vi "display.vi"() -> ()   [LabVIEW 2018]
panel:
  out "element":string
  out "Display":string[][](table)
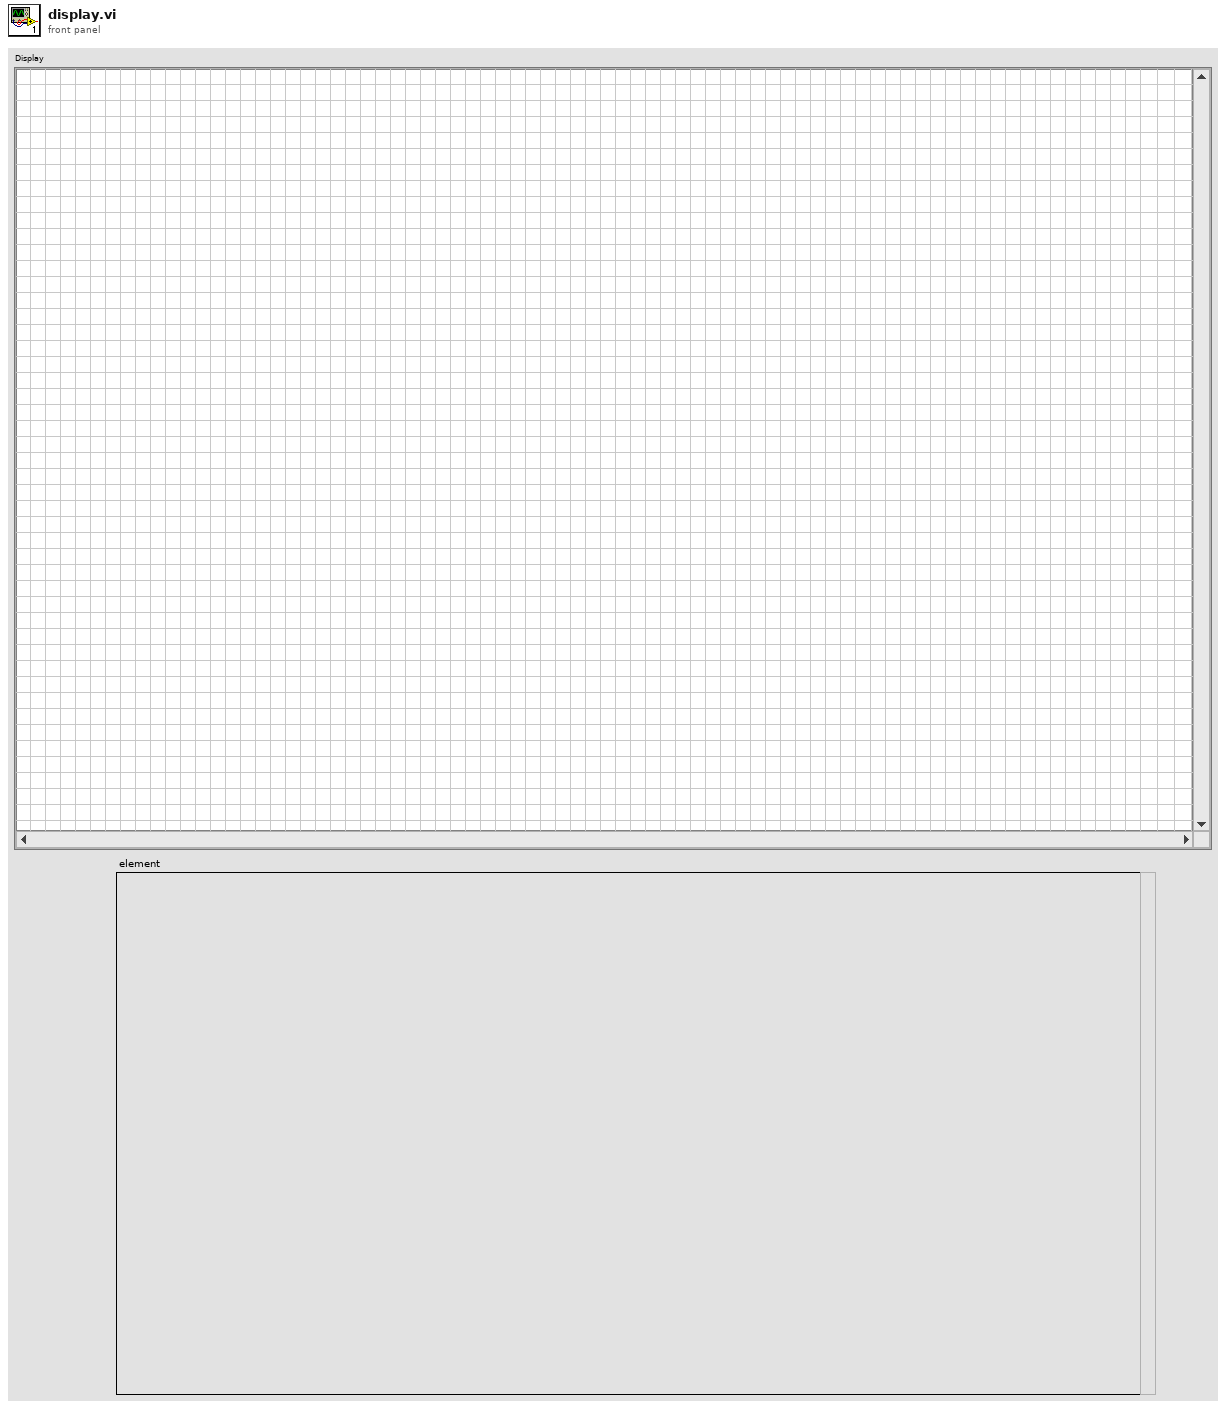
[diagram p1: front panel]
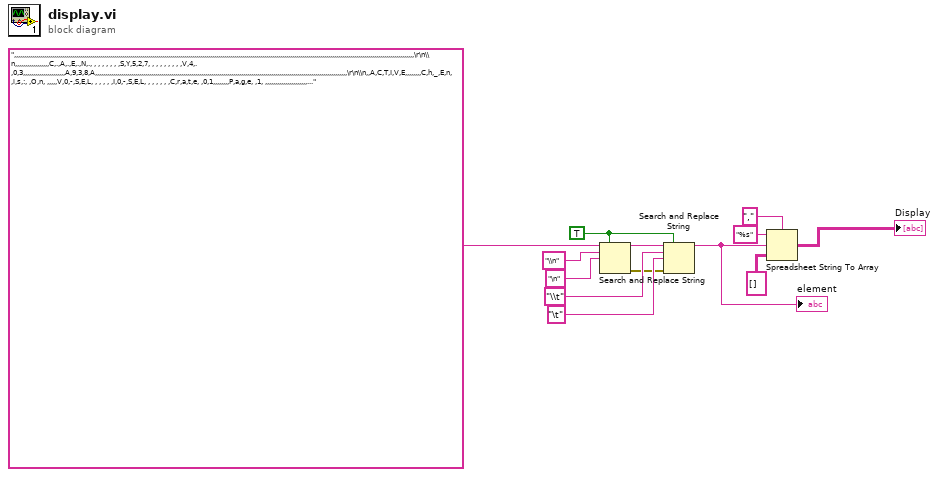
[diagram p0: block diagram]
diagram:
  w2 = TRUE ("replace all? (F)")
  n1 = Search and Replace String(replace all?=w2, input string=",,,,,,,,,,,,,,,,,,,,,,,,,,,,,,,,,,,,,,,,,,,,,,,,,,,,,,,,,,,,,,,,,,,,,,,,,,,,,,,,,,,,,,,,,,,,,,,,,,,,,,,,,,,,,,,,,,,,,,,,,,,,,,,,,,,,,,,,,,,,,,,,,,,,,,,,,,,,,,,,,,,,,,,,,,,,,,,,,,,,,,,,,,,,,,,,,,,,,,,,\r\n\\n,,,,,,,,,,,,,,,,,C,.,A,.,E,.,N,., , , , , , , ,S,Y,5,2,7, , , , , , , , ,V,4,.,0,3,,,,,,,,,,,,,,,,,,,,,A,9,3,8,A,,,,,,,,,,,,,,,,,,,,,,,,,,,,,,,,,,,,,,,,,,,,,,,,,,,,,,,,,,,,,,,,,,,,,,,,,,,,,,,,,,,,,,,,,,,,,,,,,,,,,,,,,,,,,,,,,,,,,,,,,,,,,,\r\n\\n,,A,C,T,I,V,E,,,,,,,,C,h,_,E,n, ,i,s,:, ,O,n, ,,,,,V,0,-,S,E,L, , , , , ,I,0,-,S,E,L, , , , , , ,C,r,a,t,e, ,0,1,,,,,,,,P,a,g,e, ,1, ,,,,,,,,,,,,,,,,,,,,,,,,,,,,,,,,,,,,,,,,,,,,,,,,,,,,,,,,,,,,,,,,,,,,,,,,,,,,,,,,,,,,,,,,,,,,,,,,,,,,,,,,,,,,,,,,,,,,,,,,,,,,\r\n\\n,,,,,,,,,,,,,,,,,,,,,,,,,,,,,,,,,,,,,,,,,,,,,,,,,,,,,,,,,,,,,,,,,,,,,,,,,,,,,,,,,,,,,,,,,,,,,,,,,,,,,,,,,,,,,,,,,,,,,,,,,,,,,,,,,,,,,,,,,,,,,,,,,,,,,,,,,,,,,,,,,,,,,,,,,,,,,,,,,,,,,,,,,,,,,,,,,,,,,,,,\r\n\\n, ,C,h,a,n,n,e,l, , , , , ,S,V,m,a,x, , ,R,u,p, , ,R,d,w,n, , ,T,r,i,p, ,T,r,i,p,E,x, ,P,r,O,n, ,P,r,O,f,f, ,P,o,n, , ,P,d,w,n, ,P,s,w,d, ,O,n,/,O,f,f, , ,C,h,#,,,,,,,,,,,,,,,,,,,,,,,,,,,,,,,,,,,,,,,,,,,,,,,,,,,,,,,,,,,,,,,,,,,,,,,,,,,,,,,,,,,,,,,,,,,,,,,,,,,,,,,,,,,,,,,,,,,,,,,,\r\n\\n, ,C,H,A,N,N,E,L,1,6, , , , ,2,0,0,0, , ,1,0,0, , ,1,0,0, , ,0,1,0,.,0, , , ,-,-, , , , ,0,1, , , ,0,1, , , ,O,f,f, , ,R,d,w,n, , , , , , , , , , , , , ,1,.,1,6,,,,,,,,,,,,,,,,,,,,,,,,,,,,,,,,,,,,,,,,,,,,,,,,,,,,,,,,,,,,,,,,,,,,,,,,,,,,,,,,,,,,,,,,,,,,,,,,,,,,,,,,,,,,,,,,,,,,,,,,\r\n\\n, ,C,H,A,N,N,E,L,1,7, , , , ,2,0,0,0, , ,1,0,0, , ,1,0,0, , ,0,1,0,.,0, , , ,-,-, , , , ,0,1, , , ,0,1, , , ,O,f,f, , ,R,d,w,n, , , , , , , , , , , , , ,1,.,1,7,,,,,,,,,,,,,,,,,,,,,,,,,,,,,,,,,,,,,,,,,,,,,,,,,,,,,,,,,,,,,,,,,,,,,,,,,,,,,,,,,,,,,,,,,,,,,,,,,,,,,,,,,,,,,,,,,,,,,,,,\r\n\\n, ,C,H,A,N,N,E,L,1,8, , , , ,2,0,0,0, , ,1,0,0, , ,1,0,0, , ,0,1,0,.,0, , , ,-,-, , , , ,0,1, , , ,0,1, , , ,O,f,f, , ,R,d,w,n, , , , , , , , , , , , , ,1,.,1,8,,,,,,,,,,,,,,,,,,,,,,,,,,,,,,,,,,,,,,,,,,,,,,,,,,,,,,,,,,,,,,,,,,,,,,,,,,,,,,,,,,,,,,,,,,,,,,,,,,,,,,,,,,,,,,,,,,,,,,,,\r\n\\n, ,C,H,A,N,N,E,L,1,9, , , , ,2,0,0,0, , ,1,0,0, , ,1,0,0, , ,0,1,0,.,0, , , ,-,-, , , , ,0,1, , , ,0,1, , , ,O,f,f, , ,R,d,w,n, , , , , , , , , , , , , ,1,.,1,9,,,,,,,,,,,,,,,,,,,,,,,,,,,,,,,,,,,,,,,,,,,,,,,,,,,,,,,,,,,,,,,,,,,,,,,,,,,,,,,,,,,,,,,,,,,,,,,,,,,,,,,,,,,,,,,,,,,,,,,,\r\n\\n, ,C,H,A,N,N,E,L,2,0, , , , ,2,0,0,0, , ,1,0,0, , ,1,0,0, , ,0,1,0,.,0, , , ,-,-, , , , ,0,1, , , ,0,1, , , ,O,f,f, , ,R,d,w,n, , , , , , , , , , , , , ,1,.,2,0,,,,,,,,,,,,,,,,,,,,,,,,,,,,,,,,,,,,,,,,,,,,,,,,,,,,,,,,,,,,,,,,,,,,,,,,,,,,,,,,,,,,,,,,,,,,,,,,,,,,,,,,,,,,,,,,,,,,,,,,\r\n\\n, ,C,H,A,N,N,E,L,2,1, , , , ,2,0,0,0, , ,1,0,0, , ,1,0,0, , ,0,1,0,.,0, , , ,-,-, , , , ,0,1, , , ,0,1, , , ,O,f,f, , ,R,d,w,n, , , , , , , , , , , , , ,1,.,2,1,,,,,,,,,,,,,,,,,,,,,,,,,,,,,,,,,,,,,,,,,,,,,,,,,,,,,,,,,,,,,,,,,,,,,,,,,,,,,,,,,,,,,,,,,,,,,,,,,,,,,,,,,,,,,,,,,,,,,,,,\r\n\\n, ,C,H,A,N,N,E,L,2,2, , , , ,2,0,0,0, , ,1,0,0, , ,1,0,0, , ,0,1,0,.,0, , , ,-,-, , , , ,0,1, , , ,0,1, , , ,O,f,f, , ,R,d,w,n, , , , , , , , , , , , , ,1,.,2,2,,,,,,,,,,,,,,,,,,,,,,,,,,,,,,,,,,,,,,,,,,,,,,,,,,,,,,,,,,,,,,,,,,,,,,,,,,,,,,,,,,,,,,,,,,,,,,,,,,,,,,,,,,,,,,,,,,,,,,,,\r\n\\n, ,C,H,A,N,N,E,L,2,3, , , , ,2,0,0,0, , ,1,0,0, , ,1,0,0, , ,0,1,0,.,0, , , ,-,-, , , , ,0,1, , , ,0,1, , , ,O,f,f, , ,R,d,w,n, , , , , , , , , , , , , ,1,.,2,3,,,,,,,,,,,,,,,,,,,,,,,,,,,,,,,,,,,,,,,,,,,,,,,,,,,,,,,,,,,,,,,,,,,,,,,,,,,,,,,,,,,,,,,,,,,,,,,,,,,,,,,,,,,,,,,,,,,,,,,,\r\n\\n, ,C,H,A,N,N,E,L,2,4, , , , ,2,0,0,0, , ,1,0,0, , ,1,0,0, , ,0,1,0,.,0, , , ,-,-, , , , ,0,1, , , ,0,1, , , ,O,f,f, , ,R,d,w,n, , , , , , , , , , , , , ,1,.,2,4,,,,,,,,,,,,,,,,,,,,,,,,,,,,,,,,,,,,,,,,,,,,,,,,,,,,,,,,,,,,,,,,,,,,,,,,,,,,,,,,,,,,,,,,,,,,,,,,,,,,,,,,,,,,,,,,,,,,,,,,\r\n\\n, ,C,H,A,N,N,E,L,0,0, , , , ,2,0,0,0, , ,1,0,0, , ,1,0,0, , ,0,1,0,.,0, , , ,-,-, , , , ,0,1, , , ,0,1, , , ,O,f,f, , ,R,d,w,n, , , , , , , , , , , , , ,2,.,0,0,,,,,,,,,,,,,,,,,,,,,,,,,,,,,,,,,,,,,,,,,,,,,,,,,,,,,,,,,,,,,,,,,,,,,,,,,,,,,,,,,,,,,,,,,,,,,,,,,,,,,,,,,,,,,,,,,,,,,,,,\r\n\\n, ,C,H,A,N,N,E,L,0,1, , , , ,2,0,0,0, , ,1,0,0, , ,1,0,0, , ,0,1,0,.,0, , , ,-,-, , , , ,0,1, , , ,0,1, , , ,O,f,f, , ,R,d,w,n, , , , , , , , , , , , , ,2,.,0,1,,,,,,,,,,,,,,,,,,,,,,,,,,,,,,,,,,,,,,,,,,,,,,,,,,,,,,,,,,,,,,,,,,,,,,,,,,,,,,,,,,,,,,,,,,,,,,,,,,,,,,,,,,,,,,,,,,,,,,,,\r\n\\n, ,C,H,A,N,N,E,L,0,2, , , , ,2,0,0,0, , ,1,0,0, , ,1,0,0, , ,0,1,0,.,0, , , ,-,-, , , , ,0,1, , , ,0,1, , , ,O,f,f, , ,R,d,w,n, , , , , , , , , , , , , ,2,.,0,2,,,,,,,,,,,,,,,,,,,,,,,,,,,,,,,,,,,,,,,,,,,,,,,,,,,,,,,,,,,,,,,,,,,,,,,,,,,,,,,,,,,,,,,,,,,,,,,,,,,,,,,,,,,,,,,,,,,,,,,,\r\n\\n, ,C,H,A,N,N,E,L,0,3, , , , ,2,0,0,0, , ,1,0,0, , ,1,0,0, , ,0,1,0,.,0, , , ,-,-, , , , ,0,1, , , ,0,1, , , ,O,f,f, , ,R,d,w,n, , , , , , , , , , , , , ,2,.,0,3,,,,,,,,,,,,,,,,,,,,,,,,,,,,,,,,,,,,,,,,,,,,,,,,,,,,,,,,,,,,,,,,,,,,,,,,,,,,,,,,,,,,,,,,,,,,,,,,,,,,,,,,,,,,,,,,,,,,,,,,\r\n\\n, ,C,H,A,N,N,E,L,0,4, , , , ,2,0,0,0, , ,1,0,0, , ,1,0,0, , ,0,1,0,.,0, , , ,-,-, , , , ,0,1, , , ,0,1, , , ,O,f,f, , ,R,d,w,n, , , , , , , , , , , , , ,2,.,0,4,,,,,,,,,,,,,,,,,,,,,,,,,,,,,,,,,,,,,,,,,,,,,,,,,,,,,,,,,,,,,,,,,,,,,,,,,,,,,,,,,,,,,,,,,,,,,,,,,,,,,,,,,,,,,,,,,,,,,,,,\r\n\\n, ,C,H,A,N,N,E,L,0,5, , , , ,1,8,0,0, , ,1,0,0, , ,1,0,0, , ,0,1,0,.,0, , , ,-,-, , , , ,0,1, , , ,0,1, , , ,O,f,f, , ,R,d,w,n, , , , , , , , , , , , , ,2,.,0,5,,,,,,,,,,,,,,,,,,,,,,,,,,,,,,,,,,,,,,,,,,,,,,,,,,,,,,,,,,,,,,,,,,,,,,,,,,,,,,,,,,,,,,,,,,,,,,,,,,,,,,,,,,,,,,,,,,,,,,,,\r\n\\n, ,C,H,A,N,N,E,L,0,6, , , , ,1,8,0,0, , ,1,0,0, , ,1,0,0, , ,0,1,0,.,0, , , ,-,-, , , , ,0,1, , , ,0,1, , , ,O,f,f, , ,R,d,w,n, , , , , , , , , , , , , ,2,.,0,6,,,,,,,,,,,,,,,,,,,,,,,,,,,,,,,,,,,,,,,,,,,,,,,,,,,,,,,,,,,,,,,,,,,,,,,,,,,,,,,,,,,,,,,,,,,,,,,,,,,,,,,,,,,,,,,,,,,,,,,,\r\n\\n,,,,,,,,,,,,,,,,,,,,,,,,,,,,,,,,,,,,,,,,,,,,,,,,,,,,,,,,,,,,,,,,,,,,,,,,,,,,,,,,,,,,,,,,,,,,,,,,,,,,,,,,,,,,,,,,,,,,,,,,,,,,,,,,,,,,,,,,,,,,,,,,,,,,,,,,,,,,,,,,,,,,,,,,,,,,,,,,,,,,,,,,,,,,,,,,,,,,,,,,\r\n\\n,,,,,,,,,,,,,,,,,,,,,,,,,,,,,,,,,,,,,,,,,,,,,,,,,,,,,,,,,,,,,,,,,,,,,,,,,,,,,,,,,,,,,,,,,,,,,,,,,,,,,,,,,,,,,,,,,,,,,,,,,,,,,,,,,,,,,,,,,,,,,,,,,,,,,,,,,,,,,,,,,,,,,,,,,,,,,,,,,,,,,,,,,,,,,,,,,,,,,,,,\r\n\\n,,,,,,,,,,,,,,,,,,,,,,,,,,,,,,,,,,,,,,,,,,,,,,,,,,,,,,,,,,,,,,,,,,,,,,,,,,,,,,,,,,,,,,,,,,,,,,,,,,,,,,,,,,,,,,,,,,,,,,,,,,,,,,,,,,,,,,,,,,,,,,,,,,,,,,,,,,,,,,,,,,,,,,,,,,,,,,,,,,,,,,,,,,,,,,,,,,,,,,,,\r\n\\n, ,Q,u,i,t, ,E,d,i,t, ,C,h,a,n,g,e, ,A,d,d, ,I,n,s,e,r,t, ,R,e,p,l,a,c,e, ,D,e,l,e,t,e, ,U,p,d,a,t,e, ,N,e,x,t, ,P,r,e,v, ,M,o,r,e, ,S,w,i,t,c,h,,,,,,,,,,,,,,,,,,,,,,,,,,,,,,,,,,,,,,,,,,,,,,,,,,,,,,,,,,,,,,,,,,,,,,,,,,,,,,,,,,,,,,,,,,,,,,,,,,,,,,,,,,,,,,,,,,,,,,,,,,,,,,,,\r\n\\n,,,,,,,,,,,,,,,,,,,,,,,,,,,,,,,,,,,,,,,,,,,,,,,,,,,,,,,,,,,,,,,,,,,,,,,,,,,,,,,,,,,,,,,,,,,,,,,,,,,,,,,,,,,,,,,,,,,,,,,,,,,,,,,,,,,,,,,,,,,,,,,,,,,,,,,,,,,,,,,,,,,,,,,,,,,,,,,,,,,,,,,,,,,,,,,,,,,,,,,,\r\n\\n,,,,,,,,,,,,,,,,,,,,,,,,,,,,,,,,,,,,,,,,,,,,,,,,,,,,,,,,,,,,,,,,,,,,,,,,,,,,,,,,,,,,,,,,,,,,,,,,,,,,,,,,,,,,,,,,,,,,,,,,,,,,,,,,,,,,,,,,,,,,,,,,,,,,,,,,,,,,,,,,,,,,,,,,,,,,,,,,,,,,,,,,,,,,,,,,,,,,,,,,\r\n\\n,,,,,,,,,,,,,,,,,,,,,,,,,,,,,,,,,,,,,,,,,,,,,,,,,,,,,,,,,,,,,,,,,,,,,,,,,,,,,,,,,,,,,,,,,,,,,,,,,,,,,,,,,,,,,,,,,,,,,,,,,,,,,,,,,,,,,,,,,,,,,,,,,,,,,,,,,,,,,,,,,,,,,,,,,,,,,,,,,,,,,,,,,,,,,,,,,,,,,,,,\r\n\\n,,,,,,,,,,,,,,,,,,,,,,,,,,,,,,,,,,,,,,,,,,,,,,,,,,,,,,,,,,,,,,,,,,,,,,,,,,,,,,,,,,,,,,,,,,,,,,,,,,,,,,,,,,,,,,,,,,,,,,,,,,,,,,,,,,,,,,,,,,,,,,,,,,,,,,,,,,,,,,,,,,,,,,,,,,,,,,,,,,,,,,,,,,,,,,,,,,,,,,,,\r\n\\n,,,,,,,,,,,,,,,,,,,,,,,,,,,,,,,,,,,,,,,,,,,,,,,,,,,,,,,,,,,,,,,,,,,,,,,,,,,,,,,,,,,,,,,,,,,,,,,,,,,,,,,,,,,,,,,,,,,,,,,,,,,,,,,,,,,,,,,,,,,,,,,,,,,,,,,,,,,,,,,,,,,,,,,,,,,,,,,,,,,,,,,,,,,,,,,,,,,,,,,,\r\n\\n,,,,,,,,,,,,,,,,,,,,,,,,,,,,,,,,,,,,,,,,,,,,,,,,,,,,,,,,,,,,,,,,,,,,,,,,,,,,,,,,,,,,,,,,,,,,,,,,,,,,,,,,,,,,,,,,,,,,,,,,,,,,,,,,,,,,,,,,,,,,,,,,,,,,,,,,,,,,,,,,,,,,,,,,,,,,,,,,,,,,,,,,,,,,,,,,,,,,,,,,\r\n\\n,,,,,,,,,,,,,,,,,,,,,,,,,,,,,,,,,,,,,,,,,,,,,,,,,,,,,,,,,,,,,,,,,,,,,,,,,,,,,,,,,,,,,,,,,,,,,,,,,,,,,,,,,,,,,,,,,,,,,,,,,,,,,,,,,,,,,,,,,,,,,,,,,,,,,,,,,,,,,,,,,,,,,,,,,,,,,,,,,,,,,,,,,,,,,,,,,,,,,,,,\r\n\\n,,,,,,,,,,,,,,,,,,,,,,,,,,,,,,,,,,,,,,,,,,,,,,,,,,,,,,,,,,,,,,,,,,,,,,,,,,,,,,,,,,,,,,,,,,,,,,,,,,,,,,,,,,,,,,,,,,,,,,,,,,,,,,,,,,,,,,,,,,,,,,,,,,,,,,,,,,,,,,,,,,,,,,,,,,,,,,,,,,,,,,,,,,,,,,,,,,,,,,,,\r\n\\n,,,,,,,,,,,,,,,,,,,,,,,,,,,,,,,,,,,,,,,,,,,,,,,,,,,,,,,,,,,,,,,,,,,,,,,,,,,,,,,,,,,,,,,,,,,,,,,,,,,,,,,,,,,,,,,,,,,,,,,,,,,,,,,,,,,,,,,,,,,,,,,,,,,,,,,,,,,,,,,,,,,,,,,,,,,,,,,,,,,,,,,,,,,,,,,,,,,,,,,,\r\n\\n,,,,,,,,,,,,,,,,,,,,,,,,,,,,,,,,,,,,,,,,,,,,,,,,,,,,,,,,,,,,,,,,,,,,,,,,,,,,,,,,,,,,,,,,,,,,,,,,,,,,,,,,,,,,,,,,,,,,,,,,,,,,,,,,,,,,,,,,,,,,,,,,,,,,,,,,,,,,,,,,,,,,,,,,,,,,,,,,,,,,,,,,,,,,,,,,,,,,,,,,\r\n\\n,,,,,,,,,,,,,,,,,,,,,,,,,,,,,,,,,,,,,,,,,,,,,,,,,,,,,,,,,,,,,,,,,,,,,,,,,,,,,,,,,,,,,,,,,,,,,,,,,,,,,,,,,,,,,,,,,,,,,,,,,,,,,,,,,,,,,,,,,,,,,,,,,,,,,,,,,,,,,,,,,,,,,,,,,,,,,,,,,,,,,,,,,,,,,,,,,,,,,,,,\r\n\\n,,,,,,,,,,,,,,,,,,,,,,,,,,,,,,,,,,,,,,,,,,,,,,,,,,,,,,,,,,,,,,,,,,,,,,,,,,,,,,,,,,,,,,,,,,,,,,,,,,,,,,,,,,,,,,,,,,,,,,,,,,,,,,,,,,,,,,,,,,,,,,,,,,,,,,,,,,,,,,,,,,,,,,,,,,,,,,,,,,,,,,,,,,,,,,,,,,,,,,,,\r\n\\n,,,,,,,,,,,,,,,,,,,,,,,,,,,,,,,,,,,,,,,,,,,,,,,,,,,,,,,,,,,,,,,,,,,,,,,,,,,,,,,,,,,,,,,,,,,,,,,,,,,,,,,,,,,,,,,,,,,,,,,,,,,,,,,,,,,,,,,,,,,,,,,,,,,,,,,,,,,,,,,,,,,,,,,,,,,,,,,,,,,,,,,,,,,,,,,,,,,,,,,,\r\n\\n,,,,,,,,,,,,,,,,,,,,,,,,,,,,,,,,,,,,,,,,,,,,,,,,,,,,,,,,,,,,,,,,,,,,,,,,,,,,,,,,,,,,,,,,,,,,,,,,,,,,,,,,,,,,,,,,,,,,,,,,,,,,,,,,,,,,,,,,,,,,,,,,,,,,,,,,,,,,,,,,,,,,,,,,,,,,,,,,,,,,,,,,,,,,,,,,,,,,,,,,\r\n\\n,,,,,,,,,,,,,,,,,,,,,,,,,,,,,,,,,,,,,,,,,,,,,,,,,,,,,,,,,,,,,,,,,,,,,,,,,,,,,,,,,,,,,,,,,,,,,,,,,,,,,,,,,,,,,,,,,,,,,,,,,,,,,,,,,,,,,,,,,,,,,,,,,,,,,,,,,,,,,,,,,,,,,,,,,,,,,,,,,,,,,,,,,,,,,,,,,,,,,,,,\r\n\\n,,,,,,,,,,,,,,,,,,,,,,,,,,,,,,,,,,,,,,,,,,,,,,,,,,,,,,,,,,,,,,,,,,,,,,,,,,,,,,,,,,,,,,,,,,,,,,,,,,,,,,,,,,,,,,,,,,,,,,,,,,,,,,,,,,,,,,,,,,,,,,,,,,,,,,,,,,,,,,,,,,,,,,,,,,,,,,,,,,,,,,,,,,,,,,,,,,,,,,,,\r\n\\n" ("format string"), search string="\\n" ("format string"), replace string="\n" ("format string")) -> (result string=w5:string, error out=w3:errorcluster)  [unwired: 4 in, 2 out]
  n2 = Search and Replace String(replace all?=w2, input string=w5, search string="\\t" ("input string"), replace string="\t" ("input string"), error in=w3) -> (result string=w4:string)  [unwired: 3 in, 3 out]
  "element" <- w4
  n3 = Spreadsheet String To Array(delimiter (Tab)=",", format string="%s", spreadsheet string=w4, array type (2D Dbl)=string[][] [] ("Display")) -> (array=→"Display":string[][])
